vi "create executor.vi"(8 "error in":errorcluster, 9 "default pool size":i32, 11 "launcher ref":refnum<vi>) -> (0 "error out":errorcluster, 3 "executor reference":T1)   [LabVIEW 2013, in "thread pool.lvclass"]
uses:
  thread pool.lvclass
  task/strict executor reference.ctl
  task/task.lvclass
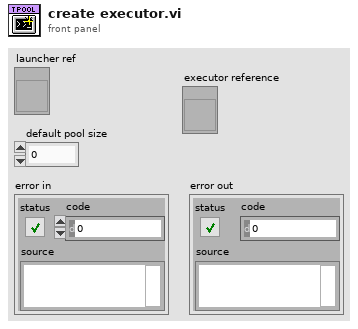
[diagram p1: front panel]
types:
  T1 = typedef "thread pool.lvclass/strict executor reference.ctl" = refnum<vi>
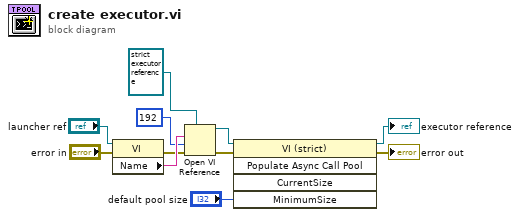
[diagram p0: block diagram]
diagram:
  n1 = property class="VI"(reference="launcher ref", error in="error in") -> (error out=w8:errorcluster, "Name"=w11:string)  [unwired: 1 out]
  n2 = Open VI Reference(type specifier VI Refnum (for type only)=T1 refnum ("executor reference"), vi path=w11, options=192, error in (no error)=w8) -> (vi reference=w4:T1, error out=w7:errorcluster)  [unwired: 2 in]
  n3 = invoke class="VI (strict)" method="Populate Async Call Pool"(reference=w4, error in=w7, "MinimumSize"="default pool size") -> (reference out=→"executor reference":T1, error out=→"error out":errorcluster)  [unwired: 2 in, 3 out]
